vi "flow-gen.io-compare-out.vi"(7 "Step Label":string, 9 "File":string, 10 "stepPointer (False Cond.)":string, 11 "Device Sensor Params":T1={"Input"="ain", "Comparison"=">=", "Setpoint"=0.0}) -> (3 "Step out":T3)   [LabVIEW 2024]
uses:
  controls/UiStepBuilder.ctl
  controls/type.step-builder.ctl
  controls/UiDeviceSensorParams.ctl
  controls/UiDeviceSensorEquality.ctl
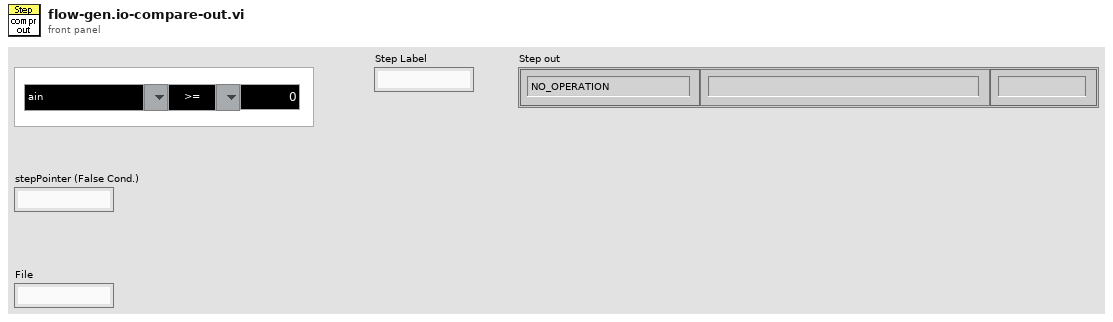
[diagram p1: front panel]
types:
  T1 = typedef "UiDeviceSensorParams.ctl" = cluster{"Input":string, "Comparison":T2, "Setpoint":dbl}
  T2 = typedef "UiDeviceSensorEquality.ctl" = string
  T3 = typedef "UiStepBuilder.ctl" = cluster{"Step Function":T4, "ParamString":string, "Step Label":string}
  T4 = typedef "type.step-builder.ctl" = enum16{"NO_OPERATION", "DELAY-JUMP", "DELAY", "JUMP", "COMPLETE", "SCHEDULER", "IRR-CHECK", "UNIT-CHECK", "UNIT-SAMPLE", "UNIT-DOSE", "LOG-REPORT", "LOG-MESSAGE", "IO-READ", "IO-READ-MANY", "IO-WRITE", "IO-COMPARE-OUT", "IO-COMPARE-IN", "PROC-START", "PROC-STOP", "PROC-LOAD", "PROC-IS-COMPLETED", "RECORD-MOVE", "GET-RH", "GET-UV", "GET-WD", "GET-WS", "OCS-CHECK", "OCS-RECORD"}
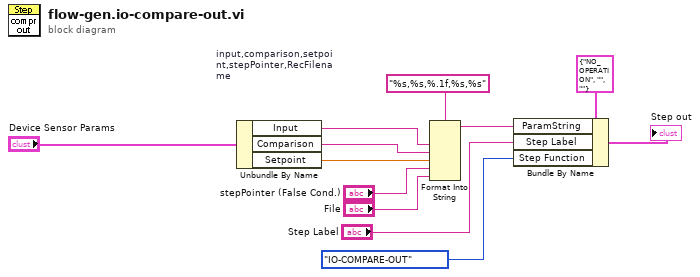
[diagram p0: block diagram]
diagram:
  w10 = "%s,%s,%.1f,%s,%s"  # input,comparison,setpoint,stepPointer,RecFilename
  n1 = Unbundle By Name("Device Sensor Params") -> ("Input"=w4:string, "Comparison"=w3:T2, "Setpoint"=w2:dbl)
  n2 = Format Into String(format string=w10, w4, w3, w2, "stepPointer (False Cond.)", "File") -> (resulting string=w9:string)  [unwired: 2 in, 1 out]
  n3 = Bundle By Name(cluster=T3 {"Step Function"=enum."NO_OPERATION", "ParamString"="", "Step Label"=""} ("FlowModeConstant 2"), "ParamString"=w9, "Step Label"="Step Label", "Step Function"=type.step-builder."IO-COMPARE-OUT") -> (→"Step out":T3)
